vi "configuration UI.vi"() -> ()   [LabVIEW 2020, in "DDS editor node.lvclass"]
uses:
  dds editor node.lvclass
  <vilib>/NI/Configuration Framework/Node/NodeRef.ctl
  <vilib>/NI/Configuration Framework/Node/NISE_CEF_Node.lvclass
  <vilib>/NI/AMC/Message Queue.ctl
  <vilib>/NI/AMC/Message.ctl
  <vilib>/NI/Tools/Keyed Array/KeyedArray.ctl
  <vilib>/NI/Configuration Framework/Node/UserEventRef.ctl
  <vilib>/NI/Configuration Framework/Controls/EventCluster.ctl
  <vilib>/NI/DCAF UI Toolkit/Controls/Configure.ctl
  <vilib>/NI/DCAF UI Toolkit/Controls/Add.ctl
  <vilib>/NI/DCAF UI Toolkit/Controls/Remove.ctl
  <vilib>/NI/Configuration Framework/Node/StopEvent.ctl
  <vilib>/NI/Configuration Framework/Node/RefreshUIEvent.ctl
  <vilib>/NI/Configuration Framework/Node/CacheState.ctl
  <vilib>/NI/Configuration Framework/Node/NodeChangeEvent.ctl
  dds data types.ctl
  Permissions Enum.ctl
  <vilib>/NI/DCAF/Tag Editor Core/Table API/Available Tag Menu/channel action event.ctl
  <vilib>/NI/DCAF/Tag Editor Core/Table API/Available Tag Menu/dialog output action.ctl
  <vilib>/NI/Tag Bus Module Framework/channel/TBM channel.lvclass
  <vilib>/NI/Tag Bus/tag/tag descriptor.lvclass
  <vilib>/NI/DCAF/Tag Editor Core/Table API/Table Manager/Call Back Ref Type Def.ctl
  <vilib>/NI/DCAF/Tag Editor Core/Configuration Editor/Classes/Engine Parent/Engine Parent Editor Node.lvclass
  <vilib>/NI/DCAF/Tag Editor Core/Configuration Editor/Classes/Module editor node/module editor node.lvclass
  <vilib>/NI/DCAF/Tag Editor Core/Table API/Table Manager/references.ctl
  <vilib>/NI/DCAF/Tag Editor Core/Table API/Listbox/Multi Column Listbox.lvclass
  <vilib>/NI/Configuration Framework/NISE_CEF_TreeControl.lvlib
  <vilib>/NI/Tools/Keyed Array/Tools_KeyedArray.lvlib
  <vilib>/NI/AMC/AMC.lvlib
  <vilib>/NI/DCAF/Tag Editor Core/Table API/Table Manager/Table Manager.lvclass
  <vilib>/NI/DCAF/Tag Editor Core/Table API/Table Manager.lvlib
  <vilib>/NI/DCAF UI Toolkit/Controls/DCAF UI Elements.lvlib
panel:
  in  "user event out":refnum<user-event>
  in  "Permissions":T1
  in  "data type":T2
  in  "node change":T3
  in  "cache state":T4
  in  "refresh UI":T5
  in  "stop event":T6
  in  "Tab Control":enum32{"Static Configuration"}(tab)
  in  "Remove Button":T7
  in  "Add Button":T8
  in  "Table":i32(listbox)
  in  "settings":T9
  in  "user event":T10
  in  "main queue":T11
  in  "node ref":T12
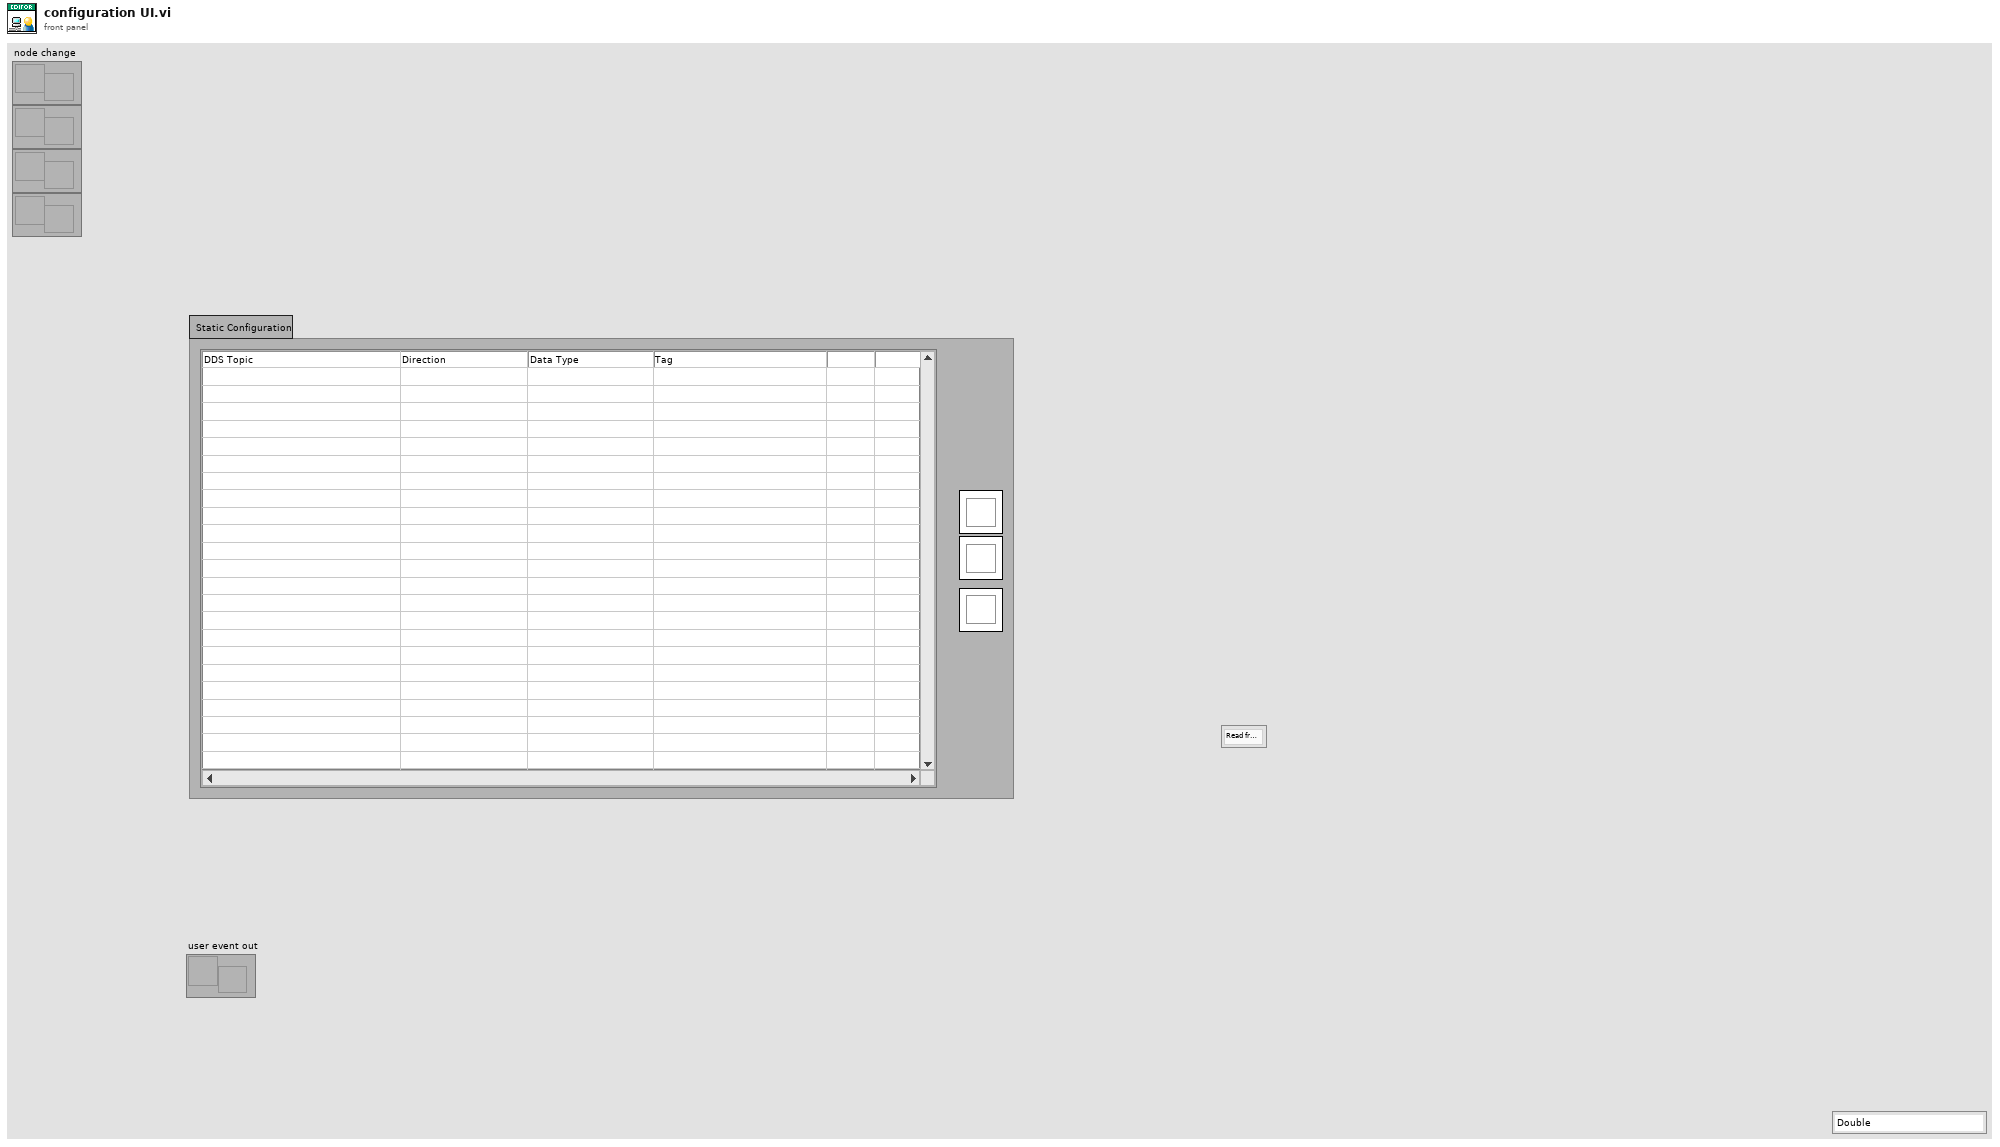
[diagram p1: front panel]
types:
  T1 = typedef "DDS editor node.lvclass/Permissions Enum.ctl" = enum16{"Read from DDS", "Write to DDS"}
  T2 = typedef "DDS editor node.lvclass/dds data types.ctl" = enum16{"Double", "Single", "I64", "I32", "I16", "I8", "U64", "U32", "U16", "U8", "Boolean", "String"}
  T3 = typedef "NISE_CEF_Node.lvclass/NodeChangeEvent.ctl" = refnum<user-event>
  T4 = typedef "NISE_CEF_Node.lvclass/CacheState.ctl" = refnum<user-event>
  T5 = typedef "NISE_CEF_Node.lvclass/RefreshUIEvent.ctl" = refnum<user-event>
  T6 = typedef "NISE_CEF_Node.lvclass/StopEvent.ctl" = refnum<user-event>
  T7 = typedef "DCAF UI Elements.lvlib/Remove.ctl" = bool
  T8 = typedef "DCAF UI Elements.lvlib/Add.ctl" = bool
  T9 = typedef "DCAF UI Elements.lvlib/Configure.ctl" = bool
  T10 = typedef "NISE_CEF_Node.lvclass/UserEventRef.ctl" = refnum<user-event>
  T11 = typedef "AMC.lvlib/Message Queue.ctl" = refnum<queue>
  T12 = typedef "NISE_CEF_Node.lvclass/NodeRef.ctl" = refnum<data-value>
  T13 = typedef "Table Manager.lvlib/Table Manager.lvclass/references.ctl" = cluster{"stop event":T6, "refresh UI":T5, "cache state":T4, "node change":T3, "user event out":refnum<user-event>, "main queue":T11, "user event":T10}
  T14 = typedef "Table Manager.lvlib/Table Manager.lvclass/object ref.ctl" = cluster{"engine":refnum<data-value>, "Node Ref":refnum<data-value>}
  T15 = typedef "Table Manager.lvlib/Column.lvclass/Column Descriptor.ctl" = cluster{"name":string, "caption":string, "Column Type":T16, "Params":string, "AutoSizeMode":i32, "FillWeight":sgl, "MinWidth":u32, "tooltip":string, "Enum Reference":refnum<vi>, "Channel suffix":string, "Read Only":bool, "Call Back VI":T17, "DT Dependency":i32, "name dependency":i32, "data type":T18, "Custom Column":refnum<class "Column.lvclass">}
  T16 = typedef "Table Manager.lvlib/Column.lvclass/Column Type.ctl" = enum16{"String", "Mapping", "Enum", "Custom"}
  T17 = typedef "Table Manager.lvlib/Table Manager.lvclass/Call Back Ref Type Def.ctl" = refnum<vi>
  T18 = typedef "tag bus.lvlib/tag descriptor.lvclass/Data Type.ctl" = enum16{"Double", "Single", "I64", "I32", "I16", "I8", "U64", "U32", "U16", "U8", "Boolean", "String", "Array of Double", "Array of Single", "Array of I64", "Array of I32", "Array of I16", "Array of I8", "Array of U64", "Array of U32", "Array of U16", "Array of U8", "Array of Boolean", "Array of String"}
  T19 = typedef "Table Manager.lvlib/Table Manager.lvclass/Table Events.ctl" = cluster{"Menu Selection":refnum<user-event>}
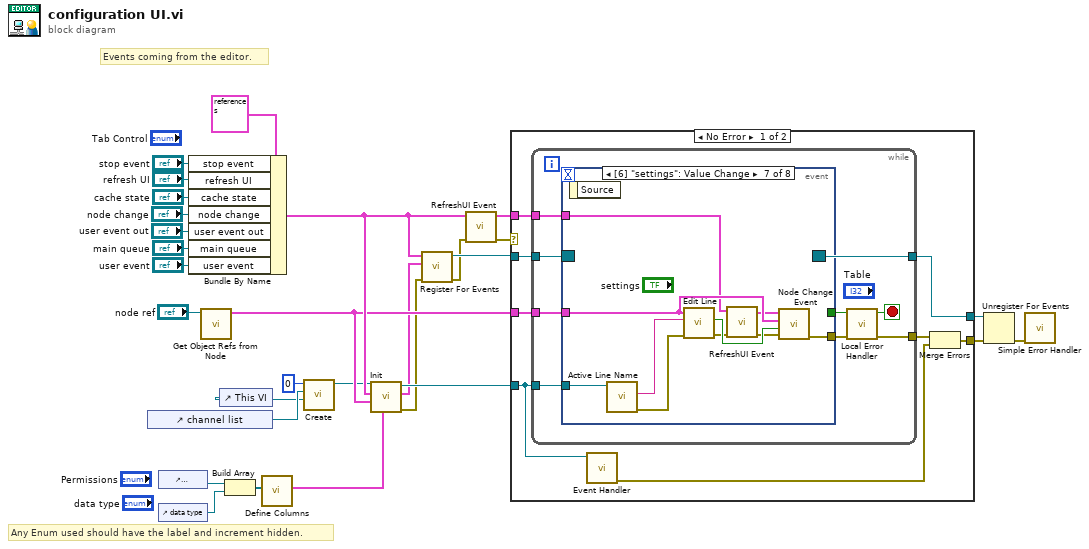
[diagram p0: block diagram]
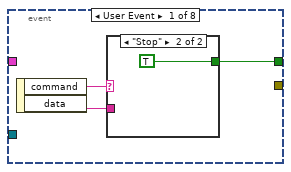
[diagram p2: hidden frame]
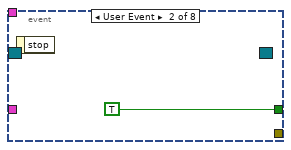
[diagram p4: hidden frame]
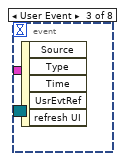
[diagram p5: hidden frame]
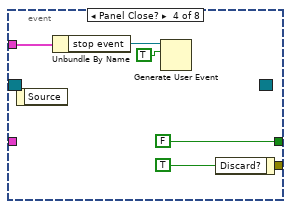
[diagram p6: hidden frame]
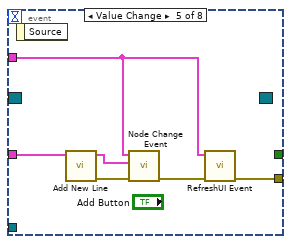
[diagram p7: hidden frame]
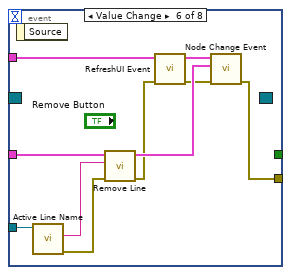
[diagram p8: hidden frame]
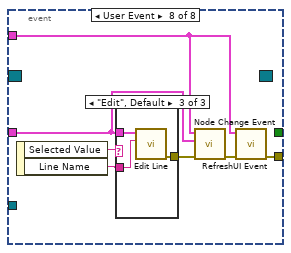
[diagram p9: hidden frame]
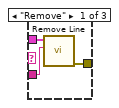
[diagram p10: hidden frame]
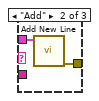
[diagram p11: hidden frame]
diagram:
  # "Any Enum used should have the label and increment hidden."
  # "Events coming from the editor."
  n1 = control-ref of="channel list"() -> (w6:refnum<vi>)
  n2 = control-ref of="Permissions"() -> (w14:refnum<vi>)
  n3 = control-ref of="data type"() -> (w2:refnum<vi>)
  n4 = Bundle By Name(cluster=T13 {"stop event"=refnum, "refresh UI"=refnum, "cache state"=refnum, "node change"=refnum, "user event out"=refnum, "main queue"=refnum, "user event"=refnum} ("References"), "stop event"="stop event", "refresh UI"="refresh UI", "cache state"="cache state", "node change"="node change", "user event out"="user event out", "main queue"="main queue", "user event"="user event") -> (w15:T13)
  n5 = call "Get Object Refs from Node.vi"("Data Value Reference in"="node ref") -> ("references"=w12:T14)  [unwired: 9 in, 1 out]
  n6 = control-ref of="This VI"() -> (w4:refnum<vi>)
  n7 = Build Array(w14, w2) -> (w13:refnum<vi>[])
  n8 = call "Define Columns.vi"("Enum Array"=w13) -> ("Column Definition"=w17:T15[])  [unwired: 10 in]
  n9 = call <vilib>:"Create.vi"("Top VI"=w4, "Listbox"=w6, "Index"=0) -> ("reference out"=w3:refnum<class "Multi Column Listbox.lvclass">)  [unwired: 7 in, 1 out]
  n10 = call-dynamic "Init.vi"("Column Descriptors"=w17, "Node object refs"=w12, "Event References"=w15, "Multi Column Listbox in"=w3) -> ("error out"=w8:errorcluster, "Table Events"=w7:T19, "Multi Column Listbox out"=w11:refnum<class "Multi Column Listbox.lvclass">)  [unwired: 5 in]
  n11 = call "Register For Events.vi"("error in"=w8, "Table Events"=w7, "References"=w15) -> ("error out"=w10:errorcluster, "Event Registration Refnum"=w18:refnum<event-registration>)  [unwired: 7 in]
  n12 = call "RefreshUI Event.vi"("error in (no error)"=w10, "References in"=w15) -> ("error out"=w9:errorcluster, "References out"=w16:T13)  [unwired: 8 in]
  n13 = case shown="No Error" w9 {
    selector: w9 -> [_ w97]
    tunnel: w18 -> [w37 w96]
    tunnel: [w36 w96] -> w29
    tunnel: [w30 w97] -> w28
    tunnel: w16 -> [w35 _]
    tunnel: w12 -> [w34 _]
    tunnel: w11 -> [w33 _]
    frame No Error {
      n14 = while {
        tunnel: w37 -> [w46]
        tunnel: [w45] -> w36
        tunnel: [w42] -> w31
        tunnel: w35 -> [w40]
        tunnel: w34 -> [w39]
        tunnel: w33 -> [w38]
        stop <- w44 stop-if-true
        n15 = event shown="[6] \"settings\": Value Change" {
          selector: w46 -> [_ _ _ _ _ _ _ _]
          dyn-events: [_ _ _ _ _ _ _ _] -> w45
          timeout: _ -> [_ _ _ _ _ _ _ _]
          tunnel: [w49 TRUE _ FALSE _ _ _ _] -> w43
          tunnel: [_ _ _ _ w57 w65 w80 w85] -> w41
          tunnel: w40 -> [_ _ _ w53 w60 w70 w73 w81]
          tunnel: w39 -> [_ _ _ _ w61 w69 w78 w82]
          tunnel: w38 -> [_ _ _ _ _ w64 w79 _]
          event User Event {
            n16 = event-data() -> ("command"=w48:string, "data"=w47:string)  [unwired: 1 in]
            n17 = case shown="\"Stop\"" w48 {
              tunnel: [_ TRUE] -> w49
              tunnel: w47 -> [_ _]
              frame Default {
              }
              frame "Stop" {
              }
            }
          }
          event User Event {
            n18 = event-data() -> ()  [unwired: 1 in, 1 out]
          }
          event User Event {
            n19 = event-data() -> ()  [unwired: 1 in, 5 out]
          }
          event Panel Close? {
            n20 = event-data() -> ()  [unwired: 1 in, 1 out]
            n21 = Unbundle By Name(w53) -> ("stop event"=w52:T6)
            n22 = Generate User Event(user event=w52, event data cluster=TRUE ("event data")) -> ()  [unwired: 2 in, 2 out]
            n23 = event-data("Discard?"=TRUE) -> ()  [unwired: 1 in, 1 out]
          }
          event Value Change {
            n24 = event-data() -> ()  [unwired: 1 in, 1 out]
            n25 = call "Add New Line.vi"("objects"=w61) -> ("error out"=w59:errorcluster)  [unwired: 9 in, 1 out]
            n26 = call "Node Change Event.vi"("error in (no error)"=w59, "objects"=w61, "References in"=w60) -> ("error out"=w58:errorcluster)  [unwired: 8 in]
            n27 = call "RefreshUI Event.vi"("error in (no error)"=w58, "References in"=w60) -> ("error out"=w57:errorcluster)  [unwired: 8 in, 1 out]
          }
          event Value Change {
            n28 = event-data() -> ()  [unwired: 1 in, 1 out]
            n29 = call-dynamic "Active Line Name.vi"("Multi Column Listbox in"=w64) -> ("error out"=w62:errorcluster, "Active Line Name"=w63:string)  [unwired: 8 in, 1 out]
            n30 = call "Remove Line.vi"("error in"=w62, "Active Line Name"=w63, "Objects"=w69) -> ("error out"=w66:errorcluster)  [unwired: 8 in]
            n31 = call "RefreshUI Event.vi"("error in (no error)"=w66, "References in"=w70) -> ("error out"=w68:errorcluster, "References out"=w67:T13)  [unwired: 8 in]
            n32 = call "Node Change Event.vi"("error in (no error)"=w68, "objects"=w69, "References in"=w67) -> ("error out"=w65:errorcluster)  [unwired: 8 in]
          }
          event Value Change {
            n33 = event-data() -> ()  [unwired: 1 in, 1 out]
            n34 = call-dynamic "Active Line Name.vi"("Multi Column Listbox in"=w79) -> ("error out"=w76:errorcluster, "Active Line Name"=w77:string)  [unwired: 8 in, 1 out]
            n35 = call "Edit Line.vi"("error in"=w76, "Line Name"=w77, "References"=w78) -> ("error out"=w74:errorcluster, "change?"=w75:bool)  [unwired: 7 in]
            n36 = call "RefreshUI Event.vi"("error in (no error)"=w74, "References in"=w73) -> ("error out"=w71:errorcluster, "References out"=w72:T13)  [unwired: 8 in]
            n37 = call "Node Change Event.vi"("error in (no error)"=w71, "Send"=w75, "objects"=w78, "References in"=w72) -> ("error out"=w80:errorcluster)  [unwired: 7 in]
          }
          event User Event {
            n38 = event-data() -> ("Selected Value"=w87:string, "Line Name"=w84:string)  [unwired: 1 in]
            n39 = case shown="\"Edit\", Default" w87 {
              tunnel: w84 -> [w90 _ w95]
              tunnel: w82 -> [w89 w92 w94]
              tunnel: [w88 w91 w93] -> w83
              frame "Remove" {
                n40 = call "Remove Line.vi"("Active Line Name"=w90, "Objects"=w89) -> ("error out"=w88:errorcluster)  [unwired: 9 in]
              }
              frame "Add" {
                n41 = call "Add New Line.vi"("objects"=w92) -> ("error out"=w91:errorcluster)  [unwired: 9 in, 1 out]
              }
              frame "Edit", Default {
                n42 = call "Edit Line.vi"("Line Name"=w95, "References"=w94) -> ("error out"=w93:errorcluster)  [unwired: 8 in, 1 out]
              }
            }
            n43 = call "Node Change Event.vi"("error in (no error)"=w83, "objects"=w82, "References in"=w81) -> ("error out"=w86:errorcluster)  [unwired: 8 in]
            n44 = call "RefreshUI Event.vi"("error in (no error)"=w86, "References in"=w81) -> ("error out"=w85:errorcluster)  [unwired: 8 in, 1 out]
          }
        }
        n45 = call "Local Error Handler.vi"("error in"=w41, "Stop in"=w43) -> ("error out"=w42:errorcluster, "Stop out"=w44:bool)  [unwired: 8 in]
      }
      n46 = call-dynamic "Event Handler.vi"("Listbox in"=w33) -> ("error out"=w32:errorcluster)  [unwired: 9 in, 1 out]
      n47 = Merge Errors(w31, w32) -> (w30:errorcluster)
    }
    frame Error {
    }
  }
  n48 = Unregister For Events(event registration refnum=w29, error in=w28) -> (error out=w27:errorcluster)
  n49 = call <vilib>:"Simple Error Handler.vi"("error in (no error)"=w27) -> ()  [unwired: 4 in, 5 out]
